vi "teardown.vi"(8 "error in":errorcluster, 11 "camera handle":u64) -> (0 "error out":errorcluster)   [LabVIEW 2019, in "PICam.lvlib"]
uses:
  PICam.lvlib
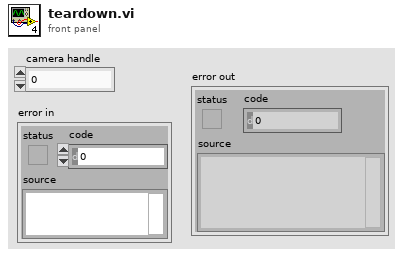
[diagram p1: front panel]
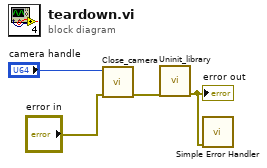
[diagram p0: block diagram]
diagram:
  n1 = call "Close_camera.vi"("error in"="error in", "camera handle in"="camera handle") -> ("error out"=w3:errorcluster)  [unwired: 9 in]
  n2 = call "Uninit_library.vi"("error in"=w3) -> ("error out"=w4:errorcluster)  [unwired: 10 in]
  "error out" <- w4
  n3 = call <vilib>:"Simple Error Handler.vi"("error in (no error)"=w4) -> ()  [unwired: 4 in, 5 out]
